vi "BENCH SELECTED.vi"() -> (3 "BANCO":i32)   [LabVIEW 2019]
uses:
  BenchSelector.vi
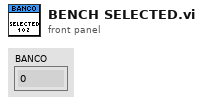
[diagram p1: front panel]
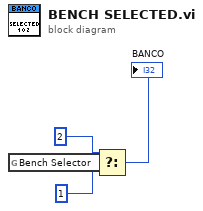
[diagram p0: block diagram]
diagram:
  n1 = global read "BenchSelector.vi" "Bench Selector"() -> (w1:bool)
  n2 = Select(t=2 ("BANCO"), s=w1, f=1 ("BANCO")) -> (s? t:f=→"BANCO":i32)
